vi "科学记数法正则表达式.vi"(8 "error in (no error)":errorcluster caption="错误输入（无错误）") -> (0 "error out":errorcluster caption="错误输出", 3 "正则表达式":string="\\[+-]?")   [LabVIEW 2012]
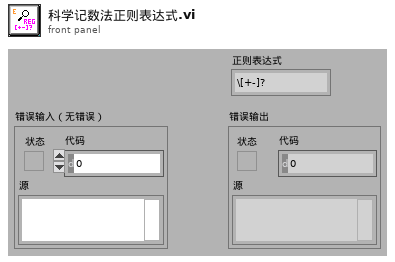
[diagram p1: front panel]
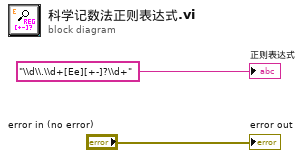
[diagram p0: block diagram]
diagram:
  "正则表达式" <- "\\d\\.\\d+[Ee][+-]?\\d+" ("正则表达式")
  "error out" <- "error in (no error)"
